vi "Create Plots.vi"(0 "Data in":T6, 5 "Display State":T1, 9 "panel":refnum<vi>) -> (15 "error out":errorcluster)   [LabVIEW 2020, in "Interactive Graph.xctl"]
uses:
  Interactive Graph.xctl
  Data.vi
  EPhys/LV Source/Work Panel VIs/Typedefs/EPhysWork-Label Position.ctl
  State.vi
  Persistent.ctl
  Plot.ctl
  Events.ctl
  Selection.ctl
  XRange.ctl
  YScale.ctl
  Cursor.ctl
  <vilib>/Analysis/baseanly.llb/Mean (DBL).vi
  <vilib>/Analysis/NI_AALBase.lvlib
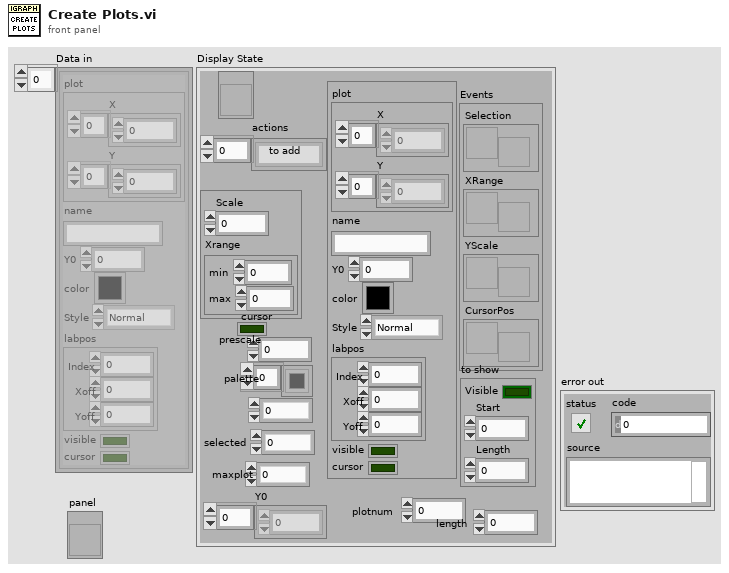
[diagram p1: front panel]
types:
  T1 = typedef "Interactive Graph.xctl/State.vi" = cluster{"ref":refnum<vi>, "actions":string[], "Persist":T2, "cursor":bool, "prescale":dbl, "palette":u32[], "colIndex":i32, "to add":T3, "Events":T5, "selected":i32, "to show":cluster{"Visible":bool, "Start":i32, "Length":i32}, "maxplot":i32, "Y0":dbl[], "plotnum":i32, "length":i32}
  T2 = typedef "Interactive Graph.xctl/Persistent.ctl" = cluster{"Scale":dbl, "Xrange":cluster{"min":dbl, "max":dbl}}
  T3 = typedef "Interactive Graph.xctl/Plot.ctl" = cluster{"plot":cluster{"X":dbl[], "Y":dbl[]}, "name":string, "Y0":dbl, "color":u32, "Style":enum16{"Normal", "Highlight", "Shadow"}, "labpos":T4, "visible":bool, "cursor":bool}
  T4 = typedef "EPhysWork-Label Position.ctl" = cluster{"Index":i32, "Xoff":dbl, "Yoff":dbl}
  T5 = typedef "Interactive Graph.xctl/Events.ctl" = cluster{"Selection":refnum<user-event>, "XRange":refnum<user-event>, "YScale":refnum<user-event>, "CursorPos":refnum<user-event>}
  T6 = typedef "Interactive Graph.xctl/Data.vi" = cluster{"plot":cluster{"X":dbl[], "Y":dbl[]}, "name":string, "Y0":dbl, "color":u32, "Style":enum16{"Normal", "Highlight", "Shadow"}, "labpos":T4, "visible":bool, "cursor":bool}[]
  T7 = cluster{"Name":string, "Color":u32, "Style":u8, "Point Style":u8, "Name Visible":bool, "Allow Drag":bool, "Cursor Mode":u32, "Plot":i32, "Index":i32, "Position":cluster{"X":dbl, "Y":dbl}, "X Scale":u32, "Y Scale":u32, "Watch Plots":i32[], "Watch All Plots":bool, "Plot Area":i32, "Label Offset":cluster{"X":dbl, "Y":dbl}}
  T8 = cluster{"Name":string, "Color":u32, "Style":u8, "Point Style":u8, "Name Visible":bool, "Allow Drag":bool, "Annotation Mode":u32, "Plot":i32, "Index":i32, "Position":cluster{"X":dbl, "Y":dbl}, "X Scale":u32, "Y Scale":u32, "Show Arrow":bool, "Lock Name":bool, "Plot Area":i32, "Label Offset":cluster{"X":dbl, "Y":dbl}}
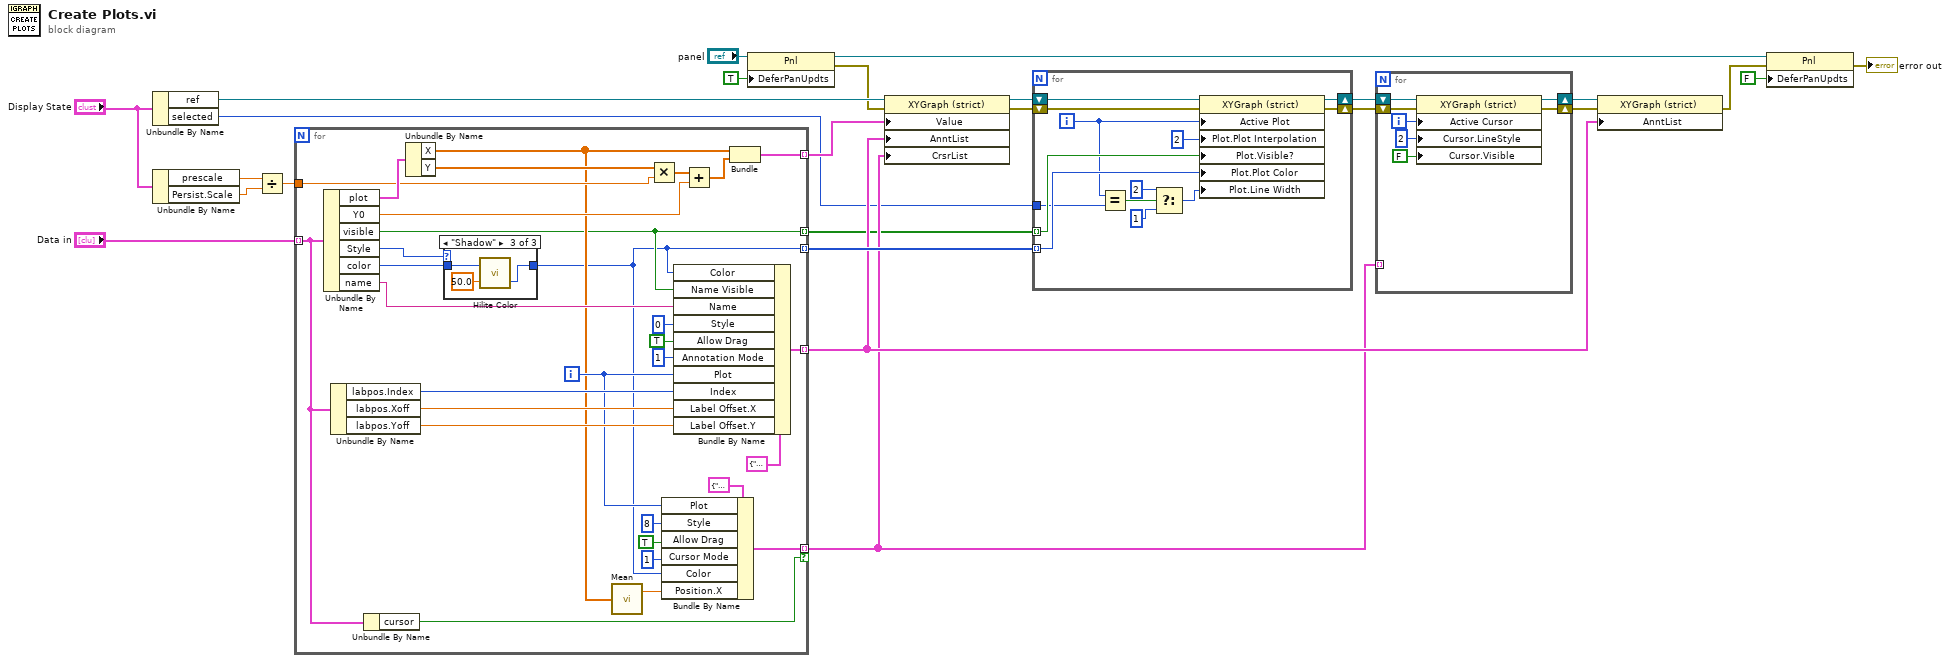
[diagram p0: block diagram]
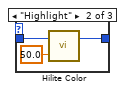
[diagram p3: hidden frame]
diagram:
  n1 = Unbundle By Name("Display State") -> ("ref"=w20:refnum<vi>, "selected"=w1:i32)
  n2 = Unbundle By Name("Display State") -> ("prescale"=w12:dbl, "Persist.Scale"=w11:dbl)
  n3 = Divide(x=w12, y=w11) -> (x/y=w10:dbl)
  n4 = for {
    tunnel: "Data in" -> [w31] mode=indexing
    tunnel: [w52] -> w19 mode=indexing
    tunnel: [w26] -> w16 mode=indexing
    tunnel: w10 -> [w53]
    tunnel: [w47] -> w9 mode=indexing
    tunnel: [w32] -> w4 mode=indexing if=w30
    tunnel: [w29] -> w3 mode=indexing
    i -> [w35]
    n5 = Unbundle By Name(w31) -> ("plot"=w55:cluster{"X":dbl[], "Y":dbl[]}, "Y0"=w42:dbl, "visible"=w29:bool, "Style"=w28:enum16{"Normal", "Highlight", "Shadow"}, "color"=w27:u32, "name"=w40:string)
    n6 = Unbundle By Name(w31) -> ("labpos.Index"=w41:i32, "labpos.Xoff"=w46:dbl, "labpos.Yoff"=w45:dbl)
    n7 = Unbundle By Name(w31) -> ("cursor"=w30:bool)
    n8 = Unbundle By Name(w55) -> ("X"=w33:dbl[], "Y"=w54:dbl[])
    n9 = case shown="\"Shadow\"" w28 {
      tunnel: [w56 w57 w60] -> w26
      tunnel: w27 -> [w56 w58 w61]
      frame "Normal", Default {
      }
      frame "Highlight" {
        n10 = call <vilib>:"Hilite Color.vi"("Percentage(30)"=50.0, "Color In"=w58) -> ("Hilite"=w57:u32)  [unwired: 1 out]
      }
      frame "Shadow" {
        n11 = call <vilib>:"Hilite Color.vi"("Percentage(30)"=50.0, "Color In"=w61) -> ("Shadow"=w60:u32)  [unwired: 1 out]
      }
    }
    n12 = call-poly <vilib>:"Mean.vi"("X"=w33) -> ("mean"=w34:dbl)  [unwired: 1 out]
    n13 = Multiply(x=w54, y=w53) -> (x*y=w43:dbl[])
    n14 = Bundle By Name(cluster=T7 {"Name"="", "Color"=0, "Style"=0, "Point Style"=0, "Name Visible"=FALSE, "Allow Drag"=FALSE, "Cursor Mode"=0, "Plot"=0, "Index"=0, "Position"={"X"=0.0, "Y"=0.0}, "X Scale"=0, "Y Scale"=0, "Watch Plots"=[], "Watch All Plots"=FALSE, "Plot Area"=0, "Label Offset"={"X"=0.0, "Y"=0.0}} ("array"), "Plot"=w35, "Style"=u8 8, "Allow Drag"=TRUE, "Cursor Mode"=u32 1, "Color"=w26, "Position.X"=w34) -> (w32:T7)
    n15 = Bundle By Name(cluster=T8 {"Name"="", "Color"=0, "Style"=0, "Point Style"=0, "Name Visible"=FALSE, "Allow Drag"=FALSE, "Annotation Mode"=0, "Plot"=0, "Index"=0, "Position"={"X"=0.0, "Y"=0.0}, "X Scale"=0, "Y Scale"=0, "Show Arrow"=FALSE, "Lock Name"=FALSE, "Plot Area"=0, "Label Offset"={"X"=0.0, "Y"=0.0}} ("new element/subarray"), "Color"=w26, "Name Visible"=w29, "Name"=w40, "Style"=u8 0, "Allow Drag"=TRUE, "Annotation Mode"=u32 1, "Plot"=w35, "Index"=w41, "Label Offset.X"=w46, "Label Offset.Y"=w45) -> (w47:T8)
    n16 = Add(x=w43, y=w42) -> (x+y=w44:dbl[])
    n17 = Bundle("X"=w33, w44) -> (w52:cluster{"X":dbl[], dbl[]})  [unwired: 1 in]
  }
  n18 = property class="Pnl"(reference="panel", "DeferPanUpdts"=TRUE ("Defer Panel Updates")) -> (reference out=w24:refnum<vi>, error out=w15:errorcluster)  [unwired: 1 in]
  n19 = property class="XYGraph (strict)"(reference=w20, error in=w15, "Value"=w19, "AnntList"=w9, "CrsrList"=w4) -> (reference out=w18:refnum<vi>, error out=w17:errorcluster)
  n20 = for {
    shift-right: [w73] -> w8
    shift-left: w17 -> [w74]
    tunnel: w16 -> [w70] mode=indexing
    shift-right: [w71] -> w7
    shift-left: w18 -> [w75]
    tunnel: w3 -> [w69] mode=indexing
    tunnel: w1 -> [w63]
    i -> [w64]
    n21 = Equal?(x=w64, y=w63) -> (x = y?=w65:bool)
    n22 = Select(t=u8 2 ("Plot.Line Width"), s=w65, f=u8 1 ("Plot.Line Width")) -> (s? t:f=w68:u8)
    n23 = property class="XYGraph (strict)"(reference=w75, error in=w74, "Active Plot"=w64, "Plot.Plot Interpolation"=u8 2, "Plot.Visible?"=w69, "Plot.Plot Color"=w70, "Plot.Line Width"=w68) -> (reference out=w71:refnum<vi>, error out=w73:errorcluster)
  }
  n24 = for {
    shift-right: [w80] -> w6
    shift-left: w8 -> [w81]
    shift-right: [w79] -> w5
    shift-left: w7 -> [w82]
    tunnel: w4 -> [_] mode=indexing
    i -> [w78]
    n25 = property class="XYGraph (strict)"(reference=w82, error in=w81, "Active Cursor"=w78, "Cursor.LineStyle"=u8 2 ("Cursor.Line Style"), "Cursor.Visible"=FALSE) -> (reference out=w79:refnum<vi>, error out=w80:errorcluster)
  }
  n26 = property class="XYGraph (strict)"(reference=w5, error in=w6, "AnntList"=w9) -> (error out=w23:errorcluster)  [unwired: 1 out]
  n27 = property class="Pnl"(reference=w24, error in=w23, "DeferPanUpdts"=FALSE ("Defer Panel Updates")) -> (error out=→"error out":errorcluster)  [unwired: 1 out]
